vi "CreateRamp.vi"(11 "ArraySize":dbl=10.0 format="%#_13g") -> (3 "Ramp Pattern":dbl[](array[numeric]))   [LabVIEW 2018]
uses:
  <vilib>/Analysis/1siggen.llb/Ramp Pattern by Samples.vi
  <vilib>/Analysis/NI_AALBase.lvlib
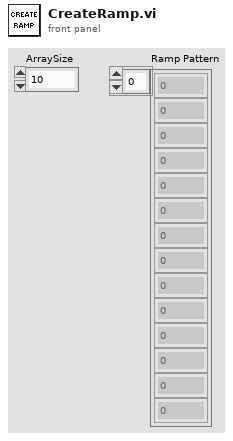
[diagram p1: front panel]
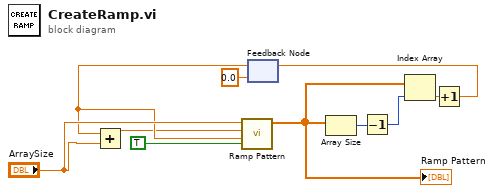
[diagram p0: block diagram]
diagram:
  n1 = feedback #1(0.0) -> (w5:dbl)
  n2 = Add(x=w5, y="ArraySize") -> (x+y=w4:dbl)
  n3 = call-poly <vilib>:"Ramp Pattern.vi"("exclude end?"=TRUE, "start"=w5, "end"=w4, "samples"="ArraySize") -> ("Ramp Pattern"=w1:dbl[])  [unwired: 6 in, 1 out]
  "Ramp Pattern" <- w1
  n4 = Array Size(array=w1) -> (size(s)=w8:i32)
  n5 = Decrement(x=w8) -> (x-1=w9:i32)
  n6 = Index Array(array=w1, index=w9) -> (element=w2:dbl)
  n7 = Increment(x=w2) -> (x+1=w10:dbl)
  n8 = feedback-in #1(w10) -> ()
